vi "EOL CAN_Reset_Memory_And_Cycle_Count GenX2.vi"(11 "CAN Network ObjHandle":T1) -> (2 "debug log":string[][](array[string]), 3 "Response Good?":bool)   [LabVIEW 2018]
uses:
  <vilib>/nican/nican.llb/xobjhandle.ctl
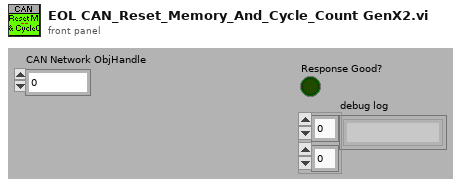
[diagram p1: front panel]
types:
  T1 = typedef "xobjhandle.ctl" = u32
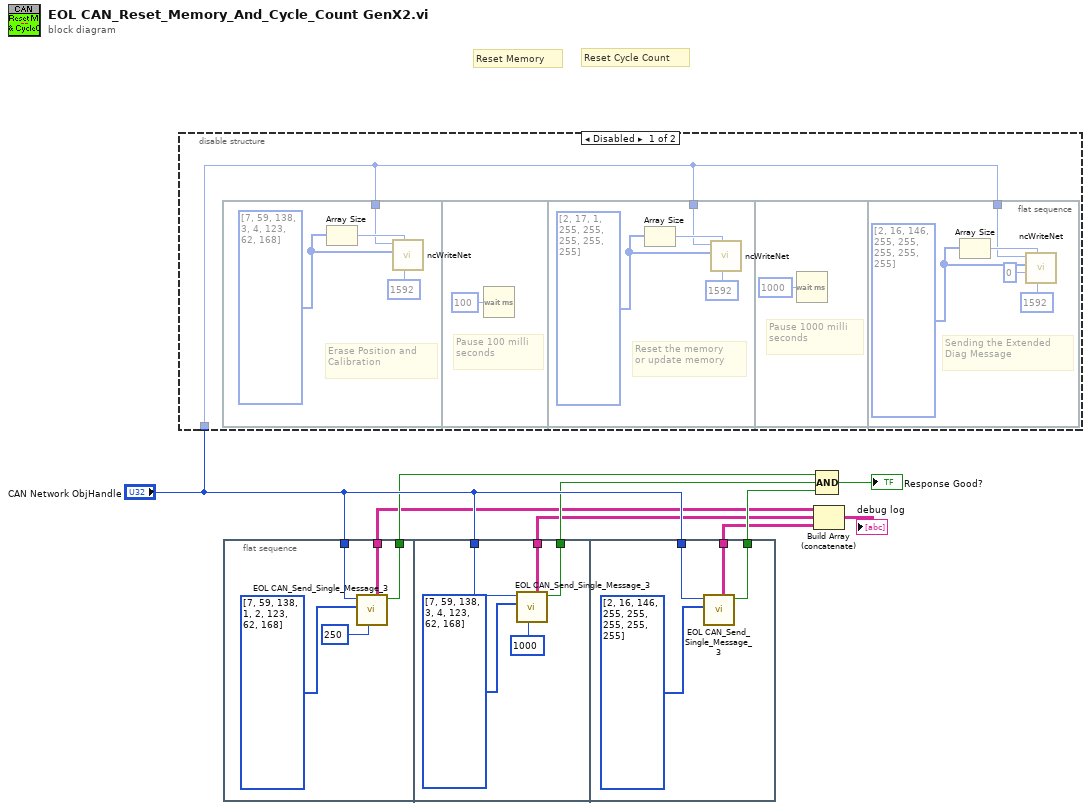
[diagram p0: block diagram]
diagram:
  # "Reset Memory"
  # "Reset Cycle Count"
  n1 = disable-structure shown="Disabled" {
    disable-tunnel: "CAN Network ObjHandle" -> [w10 _]
    frame Disabled {
      n2 = flat-sequence {
        tunnel: w10 -> [w11]
        tunnel: w10 -> [w16]
        tunnel: w10 -> [w21]
        frame #0 {
          w12 = u8[] [7, 59, 138, 3, 4, 123, 62, 168] ("Transmit Data 2")
          # "Erase Position and\nCalibration"
          n3 = Array Size(array=w12) -> (size(s)=w14:i32)
          n4 = call <vilib>:"ncWriteNet.vi"("ArbitrationId"=u32 1592 ("Transmit Id 2"), "DataLength"=w14, "Data"=w12, "ObjHandle in"=w11) -> ()  [unwired: 2 in, 2 out]
        }
        frame #1 {
          # "Pause 100 milli\nseconds"
          n5 = Wait (ms)(milliseconds to wait=u32 100) -> ()  [unwired: 1 out]
        }
        frame #2 {
          w19 = u8[] [2, 17, 1, 255, 255, 255, 255, 255] ("Transmit Data 2")
          # "Reset the memory \nor update memory"
          n6 = Array Size(array=w19) -> (size(s)=w17:i32)
          n7 = call <vilib>:"ncWriteNet.vi"("ArbitrationId"=u32 1592 ("Transmit Id 2"), "DataLength"=w17, "Data"=w19, "ObjHandle in"=w16) -> ()  [unwired: 2 in, 2 out]
        }
        frame #3 {
          # "Pause 1000 milli\nseconds"
          n8 = Wait (ms)(milliseconds to wait=u32 1000) -> ()  [unwired: 1 out]
        }
        frame #4 {
          w24 = u8[] [2, 16, 146, 255, 255, 255, 255, 255] ("Transmit Data 2")
          # "Sending the Extended\nDiag Message"
          n9 = Array Size(array=w24) -> (size(s)=w22:i32)
          n10 = call <vilib>:"ncWriteNet.vi"("ArbitrationId"=u32 1592 ("Transmit Id 2"), "DataLength"=w22, "IsRemote"=u8 0, "Data"=w24, "ObjHandle in"=w21) -> ()  [unwired: 1 in, 2 out]
        }
      }
    }
    frame Enabled {
    }
  }
  n11 = flat-sequence {
    tunnel: "CAN Network ObjHandle" -> [w30]
    tunnel: [w27] -> w8
    tunnel: [w26] -> w4
    tunnel: "CAN Network ObjHandle" -> [w35]
    tunnel: [w32] -> w7
    tunnel: [w31] -> w3
    tunnel: "CAN Network ObjHandle" -> [w39]
    tunnel: [w37] -> w6
    tunnel: [w36] -> w2
    frame #0 {
      n12 = call <userlib>:"EOL CAN_Send_Single_Message_3.vi"("Msg Wait Time"=u32 250, "Tx Msg"=u8[] [7, 59, 138, 1, 2, 123, 62, 168] ("Transmit Data 2"), "NetworkObjHandle"=w30) -> ("Response Good?"=w27:bool, "TxRx Data"=w26:string[][])  [unwired: 5 in, 2 out]
    }
    frame #1 {
      n13 = call <userlib>:"EOL CAN_Send_Single_Message_3.vi"("Msg Wait Time"=u32 1000, "Tx Msg"=u8[] [7, 59, 138, 3, 4, 123, 62, 168] ("Transmit Data 2"), "NetworkObjHandle"=w35) -> ("Response Good?"=w32:bool, "TxRx Data"=w31:string[][])  [unwired: 5 in, 2 out]
    }
    frame #2 {
      n14 = call <userlib>:"EOL CAN_Send_Single_Message_3.vi"("Tx Msg"=u8[] [2, 16, 146, 255, 255, 255, 255, 255] ("Transmit Data 2"), "NetworkObjHandle"=w39) -> ("Response Good?"=w37:bool, "TxRx Data"=w36:string[][])  [unwired: 6 in, 2 out]
    }
  }
  n15 = Build Array (concatenate)(w4, w3, w2) -> (→"debug log":string[][])
  n16 = Compound Arithmetic op=AND(w8, w7, w6) -> (→"Response Good?":bool)
